vi "String Literal Lookup.vi"(8 "Error In":errorcluster, 11 "String Literal In":string) -> (0 "Error Out":errorcluster, 3 "Resolved String":string)   [LabVIEW 2015, in "SystemLink runtime.lvclass"]
doc: "Search for template literal definitions and return definition. If definition was not found, look it up and add to lookup."
uses:
  SystemLink runtime.lvclass
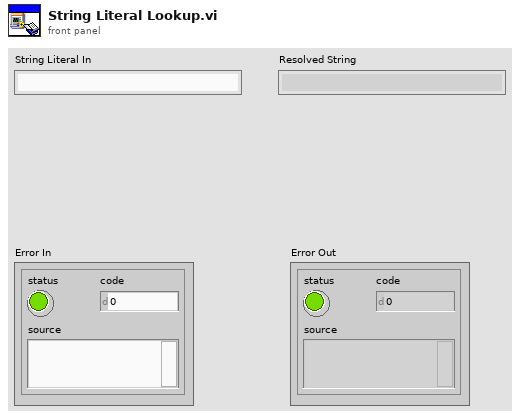
[diagram p1: front panel]
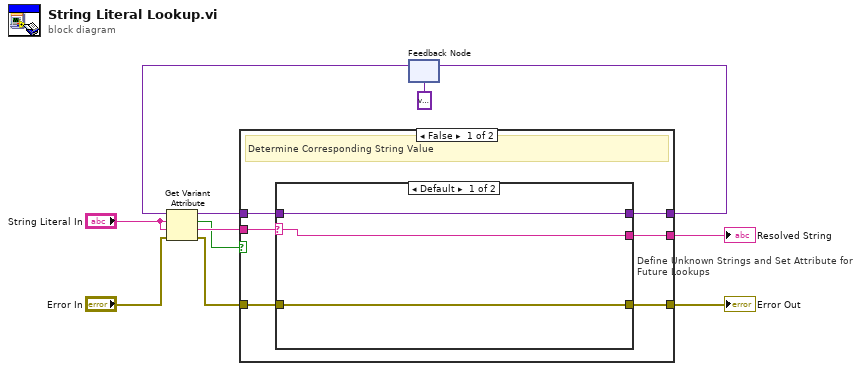
[diagram p0: block diagram]
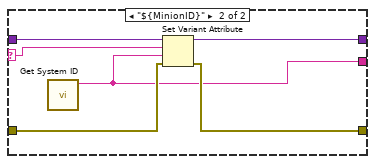
[diagram p2: hidden frame]
diagram:
  n1 = feedback #1(variant) -> (w10:variant)
  n2 = Get Variant Attribute(Variant=w10, name="String Literal In", default value (empty Variant)="String Literal In", error in="Error In") -> (duplicate Variant=w9:variant, found=w7:bool, value=w8:string, error out=w1:errorcluster)
  n3 = case shown="False" w7 {
    tunnel: w9 -> [w17 w28]
    tunnel: w8 -> [w16 w29]
    tunnel: [w12 w29] -> w6
    tunnel: [w13 w28] -> w5
    tunnel: w1 -> [w15 w27]
    tunnel: [w14 w27] -> w3
    frame False {
      # "Determine Corresponding String Value"
      n4 = case "Define Unknown Strings and Set Attribute for Future Lookups" shown="Default" w16 {
        selector: w16 -> [w18 w25]
        tunnel: w17 -> [w20 w26]
        tunnel: w15 -> [w19 w23]
        tunnel: [w19 w22] -> w14
        tunnel: [w20 w24] -> w13
        tunnel: [w18 w21] -> w12
        frame Default {
        }
        frame "${MinionID}" {
          n5 = call "Get System ID.vi"() -> ("SystemID"=w21:string)  [unwired: 11 in]
          n6 = Set Variant Attribute(Variant=w26, name=w25, value=w21, error in=w23) -> (Variant out=w24:variant, error out=w22:errorcluster)  [unwired: 1 out]
        }
      }
    }
    frame True {
      # "Pass through previously found values"
    }
  }
  "Resolved String" <- w6
  "Error Out" <- w3
  n7 = feedback-in #1(w5) -> ()
